vi "Decoder.vi"(2 "Data frame":u16[](array[numeric])) -> (16 "output cluster":T1, 19 "Kill Switch":bool)   [LabVIEW 2016]
uses:
  Typedef/Remote Control Cluster.ctl
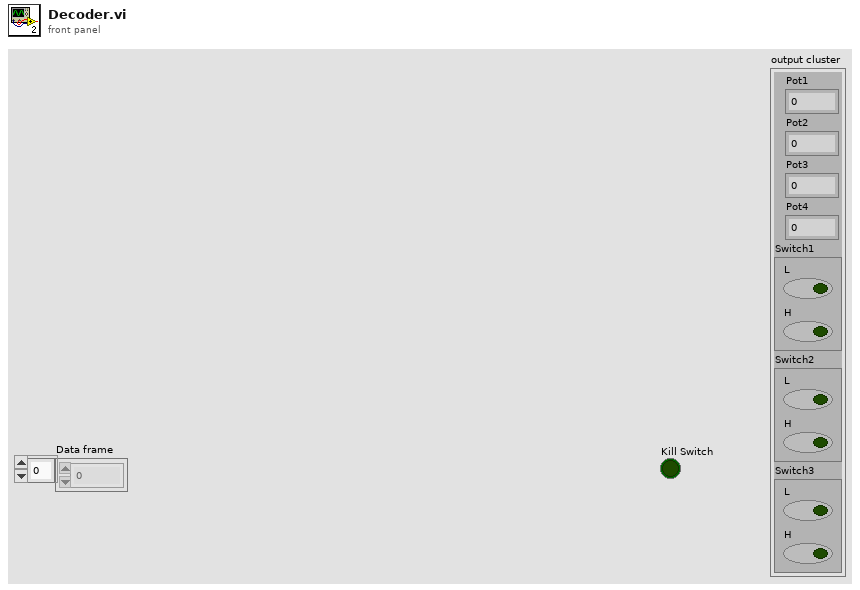
[diagram p1: front panel]
types:
  T1 = typedef "Remote Control Cluster.ctl" = cluster{"Pot1":u16, "Pot2":u16, "Pot3":u16, "Pot4":u16, "Switch1":cluster{"L":bool, "H":bool}, "Switch2":cluster{"L":bool, "H":bool}, "Switch3":cluster{"L":bool, "H":bool}}
  T2 = cluster{"Data frame[0]":u16, "Data frame[1]":u16, "Data frame[2]":u16, "Data frame[3]":u16, "Data frame[4]":u16, "Data frame[5]":u16, "Data frame[6]":u16, "Data frame[7]":u16, "Data frame[8]":u16}
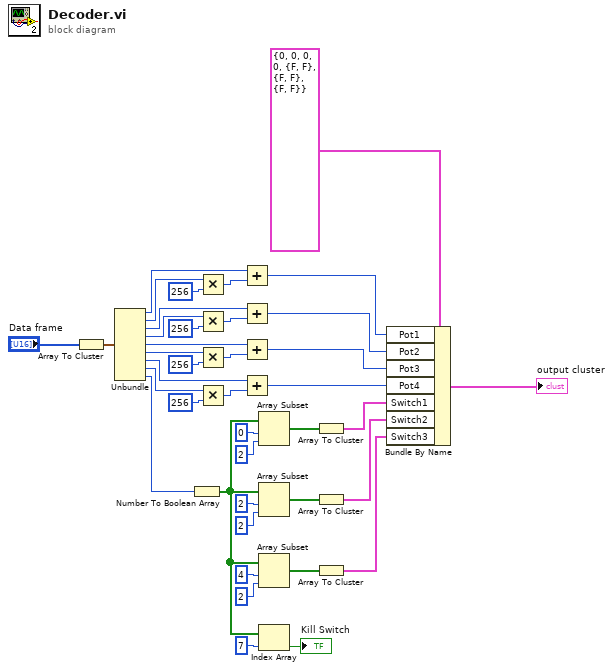
[diagram p0: block diagram]
diagram:
  n1 = Array To Cluster(array="Data frame") -> (cluster=w39:T2)
  n2 = Unbundle(w39) -> ("Data frame[0]"=w38:u16, "Data frame[1]"=w37:u16, "Data frame[2]"=w32:u16, "Data frame[3]"=w31:u16, "Data frame[4]"=w27:u16, "Data frame[5]"=w28:u16, "Data frame[6]"=w23:u16, "Data frame[7]"=w24:u16, "Data frame[8]"=w22:u16)
  n3 = Number To Boolean Array(number=w22) -> (Boolean array=w10:bool[])
  n4 = Multiply(x=w37, y=u16 256) -> (x*y=w35:u16)
  n5 = Multiply(x=w31, y=u16 256) -> (x*y=w33:u16)
  n6 = Multiply(x=w28, y=u16 256) -> (x*y=w29:u16)
  n7 = Multiply(x=w24, y=u16 256) -> (x*y=w25:u16)
  n8 = Add(x=w38, y=w35) -> (x+y=w21:u16)
  n9 = Add(x=w32, y=w33) -> (x+y=w20:u16)
  n10 = Add(x=w27, y=w29) -> (x+y=w19:u16)
  n11 = Add(x=w23, y=w25) -> (x+y=w18:u16)
  n12 = Array Subset(array=w10, index=0, length=2) -> (w7:bool[])
  n13 = Array Subset(array=w10, index=2, length=2) -> (w5:bool[])
  n14 = Array Subset(array=w10, index=4, length=2) -> (w3:bool[])
  n15 = Index Array(array=w10, index=7) -> (element=→"Kill Switch":bool)
  n16 = Array To Cluster(array=w7) -> (cluster=w6:cluster{"[0]":bool, "[1]":bool})
  n17 = Array To Cluster(array=w5) -> (cluster=w4:cluster{"[0]":bool, "[1]":bool})
  n18 = Array To Cluster(array=w3) -> (cluster=w2:cluster{"[0]":bool, "[1]":bool})
  n19 = Bundle By Name(cluster=T1 {"Pot1"=0, "Pot2"=0, "Pot3"=0, "Pot4"=0, "Switch1"={"L"=FALSE, "H"=FALSE}, "Switch2"={"L"=FALSE, "H"=FALSE}, "Switch3"={"L"=FALSE, "H"=FALSE}} ("input cluster"), "Pot1"=w21, "Pot2"=w20, "Pot3"=w19, "Pot4"=w18, "Switch1"=w6, "Switch2"=w4, "Switch3"=w2) -> (→"output cluster":T1)
